vi "JKI pwd queue manager.vi"(5 "Command (\"\")":string, 7 "Variant Data (\"\")":variant, 11 "error in (no error)":errorcluster, 12 "Mode (Get Refnum)":T1=enum."Get Refnum") -> (4 "notifier out":refnum<notifier>, 15 "error out":errorcluster)   [LabVIEW 2012]
doc: "This is the queue manager for the Please Wait Dialog\n\n<B>INPUTS</B>\n<B>Mode:</B>\nThe options are:\n< Idle>: This is operation just returns the queue value out.\nGet Refnum: This is operation just returns the queue value out.\nSend Message: This allows you to send a message to the please wait dialog. You should set a command value. Variant data is optional.\n\n<B>Command:</B>\nSpecify a text command to pass to the please wait dialog. This command must be decoded on the receiving end.\n\n<B>Variant Data:</B>\nSpecify variant data to pass with the command to the please wait dialog. This data must be decoded on the receiving end.\n\n<B>OUTPUTS</B>\n<B>Notifier Out:</B>\nThis is the queue reference that can be used to wait for messages or other external notifier functions.\n\nJKI Please Wait Dialog V1.0.2\nCopyright © 2006, James Kring, Inc.\nAll rights reserved.\n\nAuthor:\nMichael Aivaliotis\n<email: michael.aivaliotis@jameskring.com>\n<alternate email: michael@aivaliotis.com>"
uses:
  controls/JKI pwd queue data cluster.ctl
  controls/JKI pwd queue manager mode enum.ctl
panel:
  # "JKI Please Wait Dialog V1.0.2\nCopyright © 2006, James Kring, Inc.\nAll rights reserved.\n\nAuthor:\nMichael Aivaliotis\n<email: michael.aivaliotis@jameskring.com>\n<alternate email: michael@aivaliotis.com>"
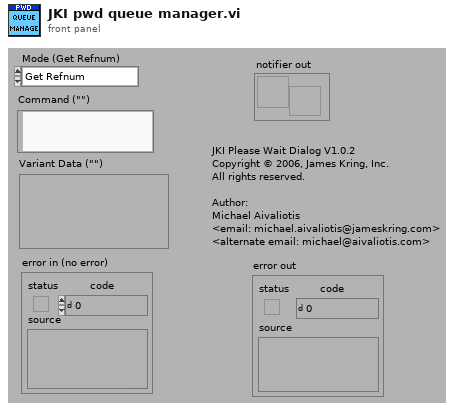
[diagram p1: front panel]
types:
  T1 = typedef "JKI pwd queue manager mode enum.ctl" = enum16{"< idle >", "Get Refnum", "Send Message"}
  T2 = typedef "JKI pwd queue data cluster.ctl" = cluster{"command":string, "variant data":variant}
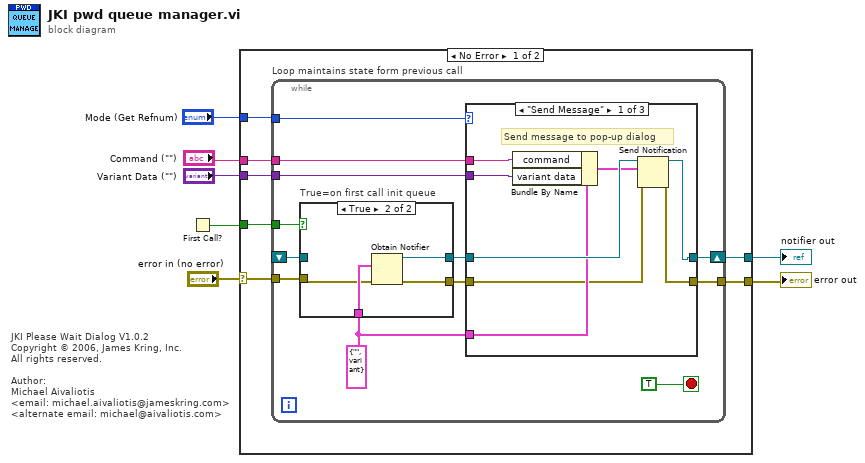
[diagram p0: block diagram]
diagram:
  # "JKI Please Wait Dialog V1.0.2\nCopyright © 2006, James Kring, Inc.\nAll rights reserved.\n\nAuthor:\nMichael Aivaliotis\n<email: michael.aivaliotis@jameskring.com>\n<alternate email: michael@aivaliotis.com>"
  n1 = First Call?() -> (First Call?: T/F=w7:bool)
  n2 = case shown="No Error" "error in (no error)" {
    selector: "error in (no error)" -> [w8 w45]
    tunnel: w7 -> [w14 _]
    tunnel: "Mode (Get Refnum)" -> [w13 _]
    tunnel: [w12 _] -> w5
    tunnel: "Command (\"\")" -> [w11 _]
    tunnel: "Variant Data (\"\")" -> [w10 _]
    tunnel: [w9 w45] -> w1
    frame No Error {
      n3 = while "Loop maintains state form previous call" {
        tunnel: w14 -> [w26]
        shift-right: [w22] -> w12
        shift-left: _ -> [w25]
        tunnel: w13 -> [w24]
        tunnel: w11 -> [w20]
        tunnel: w10 -> [w19]
        tunnel: [w17] -> w9
        tunnel: w8 -> [w16]
        stop <- TRUE stop-if-true
        w15 = T2 {"command"="", "variant data"=variant} ("Cluster")
        n4 = case "True=on first call init queue" shown="True" w26 {
          tunnel: [w40 w44] -> w23
          tunnel: w25 -> [w40 _]
          tunnel: w15 -> [_ w43]
          tunnel: [w39 w42] -> w18
          tunnel: w16 -> [w39 w41]
          frame False {
          }
          frame True {
            n5 = Obtain Notifier(notification data type=w43, error in (no error)=w41) -> (notifier out=w44:refnum<notifier>, error out=w42:errorcluster)  [unwired: 2 in, 1 out]
          }
        }
        n6 = case shown="\"Send Message\"" w24 {
          tunnel: w23 -> [w34 w36 w38]
          tunnel: [w33 w36 w38] -> w22
          tunnel: w20 -> [w32 _ _]
          tunnel: w19 -> [w31 _ _]
          tunnel: w15 -> [w30 _ _]
          tunnel: w18 -> [w28 w35 w37]
          tunnel: [w27 w35 w37] -> w17
          frame "Send Message" {
            # "Send message to pop-up dialog"
            n7 = Bundle By Name(cluster=w30, "command"=w32, "variant data"=w31) -> (w29:T2)
            n8 = Send Notification(notification=w29, notifier=w34, error in (no error)=w28) -> (notifier out=w33:refnum<notifier>, error out=w27:errorcluster)
          }
          frame "Get Refnum" {
            # "Return queue refnum"
          }
          frame "< idle >" {
            # "Idle state:\nReturn queue refnum"
          }
        }
      }
    }
    frame Error {
    }
  }
  "notifier out" <- w5
  "error out" <- w1
